vi "Pre Launch Init.vi"(11 "Measurement_Binary in":refnum<class "Measurement_Binary.lvclass">) -> (0 "error out":errorcluster, 3 "Measurement_Binary out":refnum<class "Measurement_Binary.lvclass">)   [LabVIEW 2020, in "Measurement_Binary.lvlib" / "Measurement_Binary.lvclass"]
doc: "(<B>Filename</B>: Actor Framework.lvlib:Actor.lvclass:Pre Launch Init.vi)\n\nDefines behavior that occurs after the Launch Nested Actor method is invoked but before the actor's Actor Core method begins running.\n\nBy default, this method does nothing. A descendant class may override it to define behavior."
uses:
  Measurement_Binary.lvclass
  Measurement_Binary.lvclass/Measurement_Binary.ctl
  <vilib>/ActorFramework/Actor/Actor.lvclass
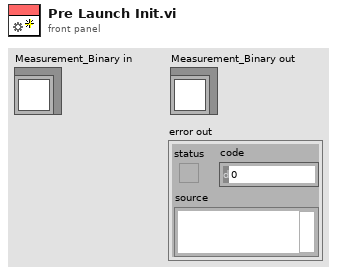
[diagram p1: front panel]
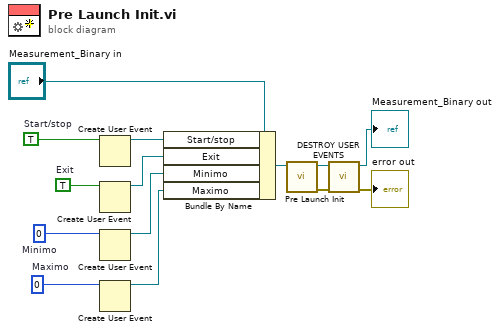
[diagram p0: block diagram]
diagram:
  w9 = u8 0  # Maximo
  w8 = u8 0  # Minimo
  w10 = TRUE  # Exit
  w11 = TRUE  # Start/stop
  n1 = Create User Event(user event datatype=w11) -> (user event=w12:refnum<user-event>)  [unwired: 1 in, 1 out]
  n2 = Create User Event(user event datatype=w10) -> (user event=w6:refnum<user-event>)  [unwired: 1 in, 1 out]
  n3 = Create User Event(user event datatype=w8) -> (user event=w7:refnum<user-event>)  [unwired: 1 in, 1 out]
  n4 = Create User Event(user event datatype=w9) -> (user event=w5:refnum<user-event>)  [unwired: 1 in, 1 out]
  n5 = Bundle By Name(cluster="Measurement_Binary in", "Start/stop"=w12, "Exit"=w6, "Minimo"=w7, "Maximo"=w5) -> (w13:refnum<class "Measurement_Binary.lvclass">)
  n6 = call-parent "Pre Launch Init.vi"("Actor in"=w13) -> ("error out"=w3:errorcluster, "Actor out"=w4:refnum<class "Measurement_Binary.lvclass">)  [unwired: 9 in]
  n7 = call "DESTROY USER EVENTS.vi"("error in (no error)"=w3, "Measurement_Binary in"=w4) -> ("error out"=→"error out":errorcluster, "Measurement_Binary out"=→"Measurement_Binary out":refnum<class "Measurement_Binary.lvclass">)  [unwired: 8 in]
